vi "Do Action.vi"(4 "error in (no error)":errorcluster, 6 "Array in":refnum<class>[](array[class]), 7 "Action in":refnum<class "Action.lvclass">) -> (0 "error out":errorcluster, 2 "Array out":refnum<class>[](array[class]), 3 "Action out":refnum<class "Action.lvclass">)   [LabVIEW 2014, in "Action.lvclass"]
uses:
  Action.lvclass
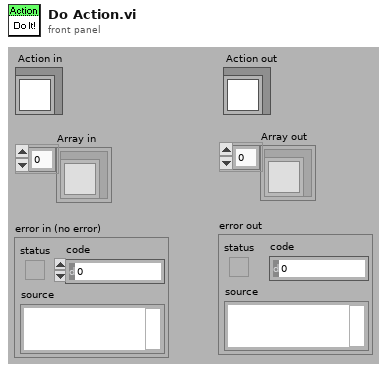
[diagram p1: front panel]
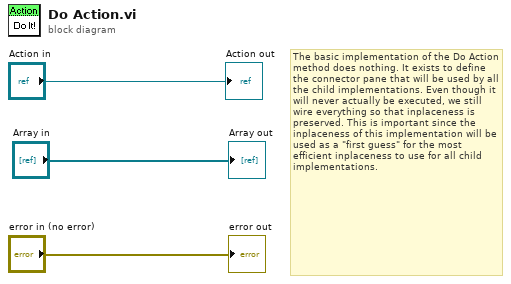
[diagram p0: block diagram]
diagram:
  # "The basic implementation of the Do Action method does nothing. It exists to define the connector pane that will be used by all the child implementations. Even though it will never actually be executed, we still wire everything so that inplaceness is preserved. This is important since the inplaceness of this implementation will be used as a \"first guess\" for the most efficient inplaceness to use for all child implementations."
  "error out" <- "error in (no error)"
  "Array out" <- "Array in"
  "Action out" <- "Action in"
